vi "Get FPGA Settings.vi"(8 "error in (no error)":errorcluster, 11 "Item Ref in":T2 format="%.0x") -> (0 "error out":errorcluster, 2 "FPGA Bitfile Settings":T1, 3 "Item Ref out":T2=18446744073709551615 format="%.0x")   [LabVIEW 2015, in "Diagnostics Addon System Explorer.lvlib"]
uses:
  Diagnostics Addon System Explorer.lvlib
  <vilib>/NI Veristand/Custom Device API/Custom Device Item Ref.ctl
  Shared/Types/FPGA Bitfile Settings.ctl
  <vilib>/NI Veristand/Custom Device API/Get Item Property (U16).vi
  Shared/SubVIs/GUID Lookup.vi
  <vilib>/NI Veristand/Custom Device API/Get Item Property (Boolean).vi
  <vilib>/NI Veristand/Custom Device API/Custom Device API.lvlib
  Shared/Diagnostics Addon Shared.lvlib
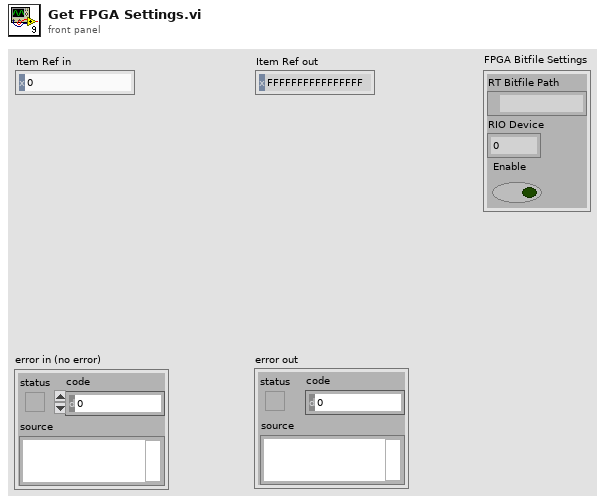
[diagram p1: front panel]
types:
  T1 = typedef "Diagnostics Addon Shared.lvlib/FPGA Bitfile Settings.ctl" = cluster{"RT Bitfile Path":path, "RIO Device":u16, "Enable":bool}
  T2 = typedef "Custom Device API.lvlib/Custom Device Item Ref.ctl" = u64
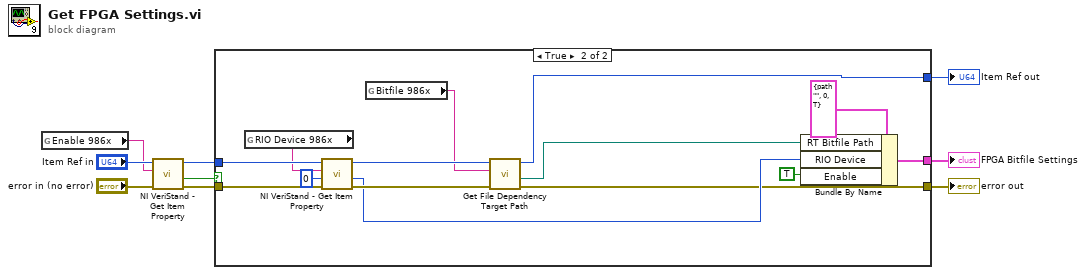
[diagram p0: block diagram]
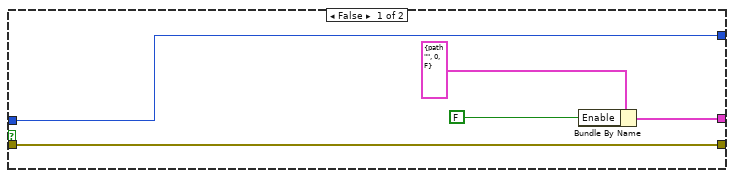
[diagram p2: hidden frame]
diagram:
  n1 = global read "GUID Lookup.vi" "Enable 986x"() -> (w1:string)
  n2 = call-poly <vilib>:"NI VeriStand - Get Item Property.vi"("error in (no error)"="error in (no error)", "Property Name"=w1, "Item Ref in"="Item Ref in") -> ("error out"=w3:errorcluster, "Value"=w4:bool, "Item Ref out"=w9:T2)  [unwired: 5 in, 1 out]
  n3 = case shown="True" w4 {
    tunnel: w9 -> [w13 w26]
    tunnel: w3 -> [w14 w28]
    tunnel: [w14 w19] -> w8
    tunnel: [w13 w16] -> w5
    tunnel: [w11 w22] -> w2
    frame False {
      n4 = Bundle By Name(cluster=T1 {"RT Bitfile Path"=path "", "RIO Device"=0, "Enable"=FALSE}, "Enable"=FALSE) -> (w11:T1)
    }
    frame True {
      n5 = global read "GUID Lookup.vi" "RIO Device 986x"() -> (w20:string)
      n6 = call-poly <vilib>:"NI VeriStand - Get Item Property.vi"("error in (no error)"=w28, "Default Value"=u16 0, "Property Name"=w20, "Item Ref in"=w26) -> ("error out"=w27:errorcluster, "Value"=w23:u16, "Item Ref out"=w18:T2)  [unwired: 4 in, 1 out]
      n7 = global read "GUID Lookup.vi" "Bitfile 986x"() -> (w17:string)
      n8 = call "Get File Dependency Target Path.vi"("error in (no error)"=w27, "Bitfile 986x"=w17, "Item Ref in"=w18) -> ("error out"=w19:errorcluster, "Target Path"=w15:path, "Item Ref out"=w16:T2)  [unwired: 5 in, 1 out]
      n9 = Bundle By Name(cluster=T1 {"RT Bitfile Path"=path "", "RIO Device"=0, "Enable"=TRUE}, "RT Bitfile Path"=w15, "RIO Device"=w23, "Enable"=TRUE) -> (w22:T1)
    }
  }
  "error out" <- w8
  "Item Ref out" <- w5
  "FPGA Bitfile Settings" <- w2
